vi "KPC101OpenLoop.vi"() -> ()   [LabVIEW 2023]
uses:
  C:/Users/fmovagharnemati/OneDrive - THORLABS Inc/Desktop/github/KPC101/Thorlabs.MotionControl.KCube.PiezoStrainGaugeCLI.dll
  Thorlabs.MotionControl.KCube.PiezoStrainGaugeCLI.dll
  C:/Users/fmovagharnemati/OneDrive - THORLABS Inc/Desktop/github/KPC101/Thorlabs.MotionControl.Controls.dll
  Thorlabs.MotionControl.Controls.dll
panel:
  in  "Voltage":dbl
  in  "Disconnect":bool
  in  "Set Voltage":bool
  in  "Serial Number":string
  in  "KCubePiezoStrainGaugeControl":refnum<k24>(container)
  # "Thorlabs Hardware: KPC - K-Cube Piezo Controller and Strain Gauge Reader\nhttps://www.thorlabs.com/thorproduct.cfm?partnumber=KPC101\n\nDescription: This VI will enable you to communicate with KPC101 in open loop mode to control Piezos via to a user set voltage. The VI will first connect and initialize the device, set a zero point, wait 10 seconds, and go in to open loop mode awaiting user command to move to a specified voltage.\n\nInstructions: \n1) Connect your KPC101  device to your PC & power the device, ensuring your stage/actutator is connected. For full device setup, the device product manual can be found on our website here. -https://www.thorlabs.com/thorproduct.cfm?partnumber=KPC101\n2) Enter the device serial number below.\n3) Ensure the device move path is clear.\n4) Click 'Run' in the LabVIEW Toolbar which will attempt a connection,set a zero point, and go into open loop mode in that order.\n5) Await for device to be be available.\n6) Input desired voltage, and press 'Set Voltage'.\n7) To end the Program click 'STOP'."
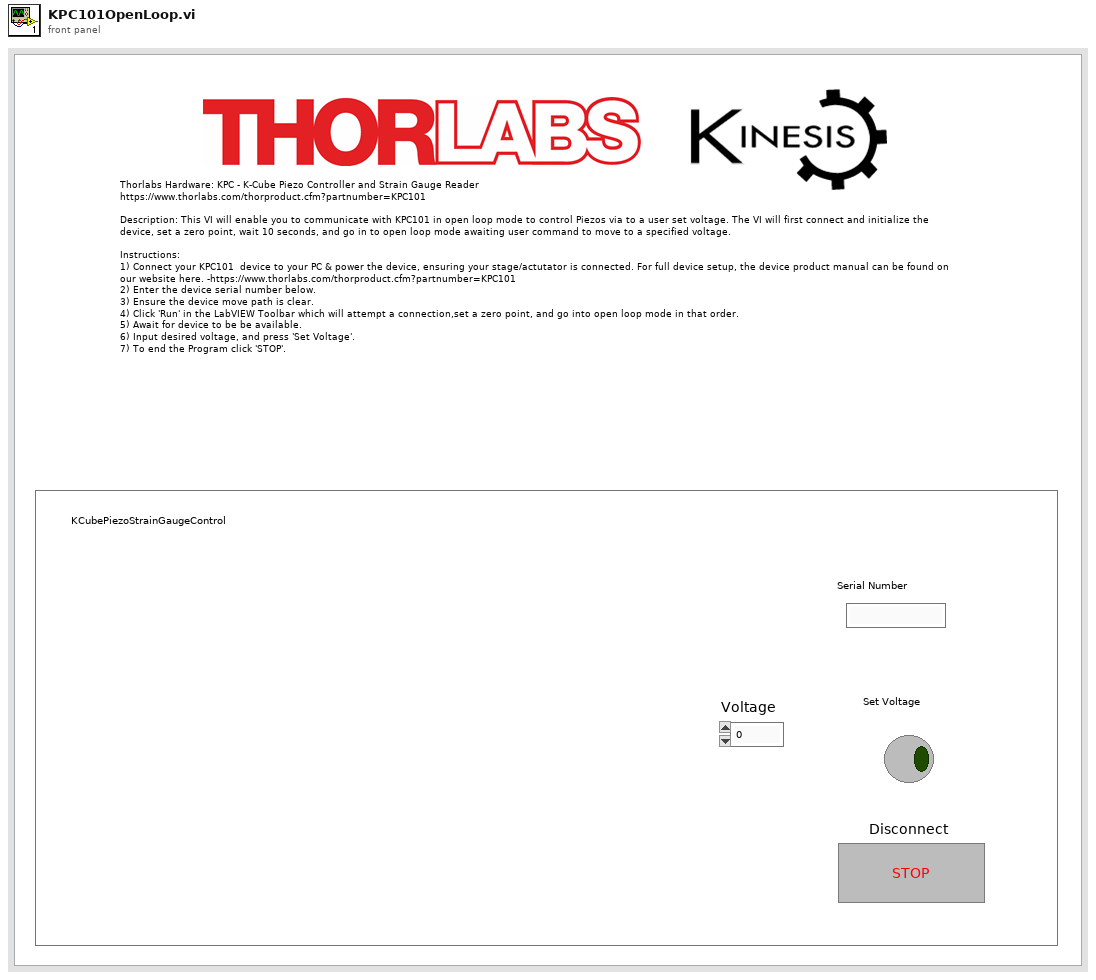
[diagram p1: front panel]
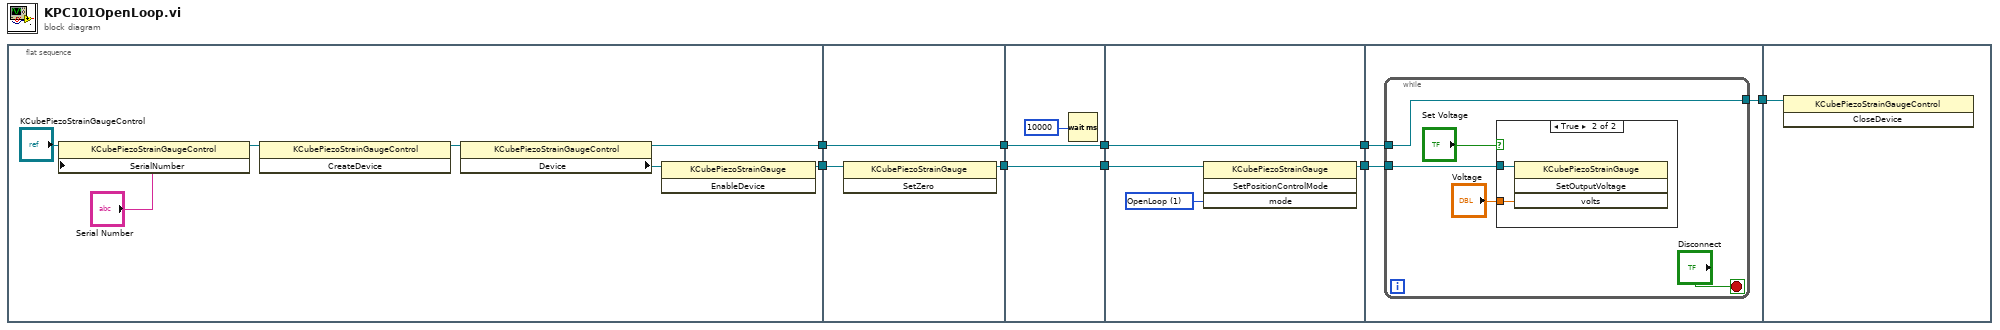
[diagram p0: block diagram]
diagram:
  n1 = flat-sequence {
    tunnel: [w11] -> w8
    tunnel: [w10] -> w7
    tunnel: [w19] -> w6
    tunnel: w8 -> [w19]
    tunnel: w7 -> [w18]
    tunnel: [w17] -> w2
    tunnel: w6 -> [w22]
    tunnel: [w22] -> w5
    tunnel: [w20] -> w3
    tunnel: w2 -> [w20]
    tunnel: w5 -> [w26]
    tunnel: [w26] -> w4
    tunnel: w3 -> [w24]
    tunnel: [w23] -> w1
    tunnel: [w29] -> w9
    tunnel: w4 -> [w28]
    tunnel: w1 -> [w27]
    tunnel: w9 -> [w37]
    frame #0 {
      n2 = property class="KCubePiezoStrainGaugeControl"(reference="KCubePiezoStrainGaugeControl", "SerialNumber"="Serial Number") -> (reference out=w15:refnum<k24>)  [unwired: 1 in, 1 out]
      n3 = invoke class="KCubePiezoStrainGaugeControl" method="CreateDevice"(reference=w15) -> (reference out=w16:refnum<k24>)  [unwired: 2 in, 2 out]
      n4 = property class="KCubePiezoStrainGaugeControl"(reference=w16) -> (reference out=w11:refnum<k24>, "Device"=w12:refnum<k24>)  [unwired: 1 in, 1 out]
      n5 = invoke class="KCubePiezoStrainGauge" method="EnableDevice"(reference=w12) -> (reference out=w10:refnum<k24>)  [unwired: 2 in, 2 out]
    }
    frame #1 {
      n6 = invoke class="KCubePiezoStrainGauge" method="SetZero"(reference=w18) -> (reference out=w17:refnum<k24>)  [unwired: 2 in, 2 out]
    }
    frame #2 {
      n7 = Wait (ms)(milliseconds to wait=u32 10000) -> ()  [unwired: 1 out]
    }
    frame #3 {
      w25 = 1 items=["OpenLoop"=1, "CloseLoop"=2, "OpenLoopSmooth"=3, "CloseLoopSmooth"=4] ("mode")
      n8 = invoke class="KCubePiezoStrainGauge" method="SetPositionControlMode"(reference=w24, "mode"=w25) -> (reference out=w23:refnum<k24>)  [unwired: 2 in, 3 out]
    }
    frame #4 {
      n9 = while {
        tunnel: [w32] -> w29
        tunnel: w28 -> [w32]
        tunnel: w27 -> [w30]
        stop <- "Disconnect" stop-if-true
        n10 = case shown="True" "Set Voltage" {
          tunnel: "Voltage" -> [_ w36]
          tunnel: w30 -> [_ w35]
          frame False {
          }
          frame True {
            n11 = invoke class="KCubePiezoStrainGauge" method="SetOutputVoltage"(reference=w35, "volts"=w36) -> ()  [unwired: 2 in, 4 out]
          }
        }
      }
    }
    frame #5 {
      n12 = invoke class="KCubePiezoStrainGaugeControl" method="CloseDevice"(reference=w37) -> ()  [unwired: 2 in, 3 out]
    }
  }
